vi "Updater.vi"(8 "Error In":errorcluster, 10 "This VI":refnum<vi>, 11 "Silent Error":bool) -> (0 "Error Out":errorcluster, 1 "Full command":string, 2 "File Version Info":string)   [LabVIEW 2016]
panel:
  out "standard output":string
  out "standard error":string
  out "return code":i32
  out "Application:Kind":T1(ring)
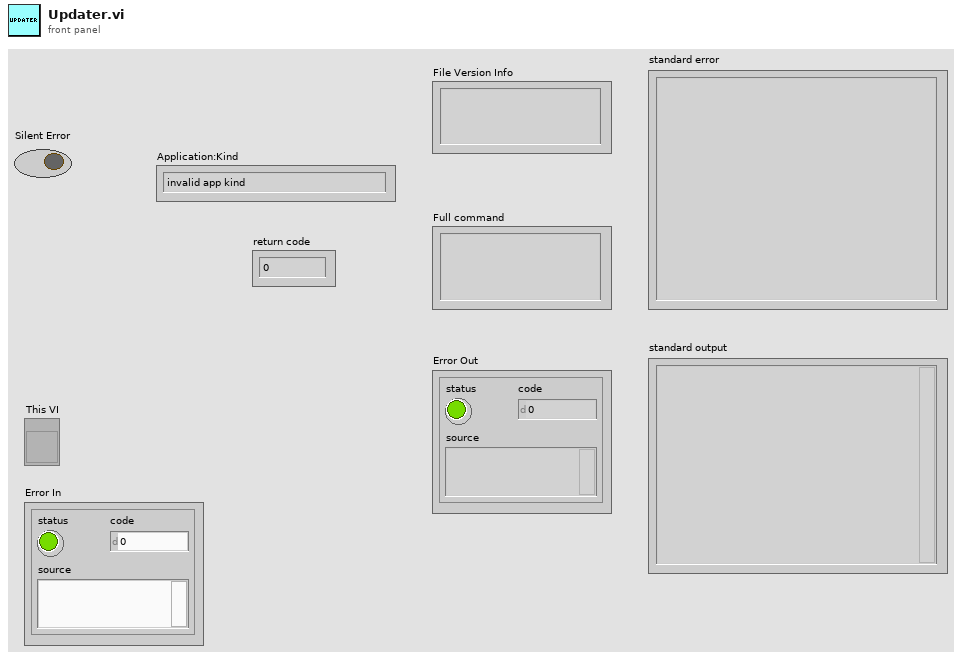
[diagram p1: front panel]
types:
  T1 = enum32{"invalid app kind", "Development System", "Run Time System", "Student Edition", "Embedded LabVIEW", "Evaluation", "Custom"}
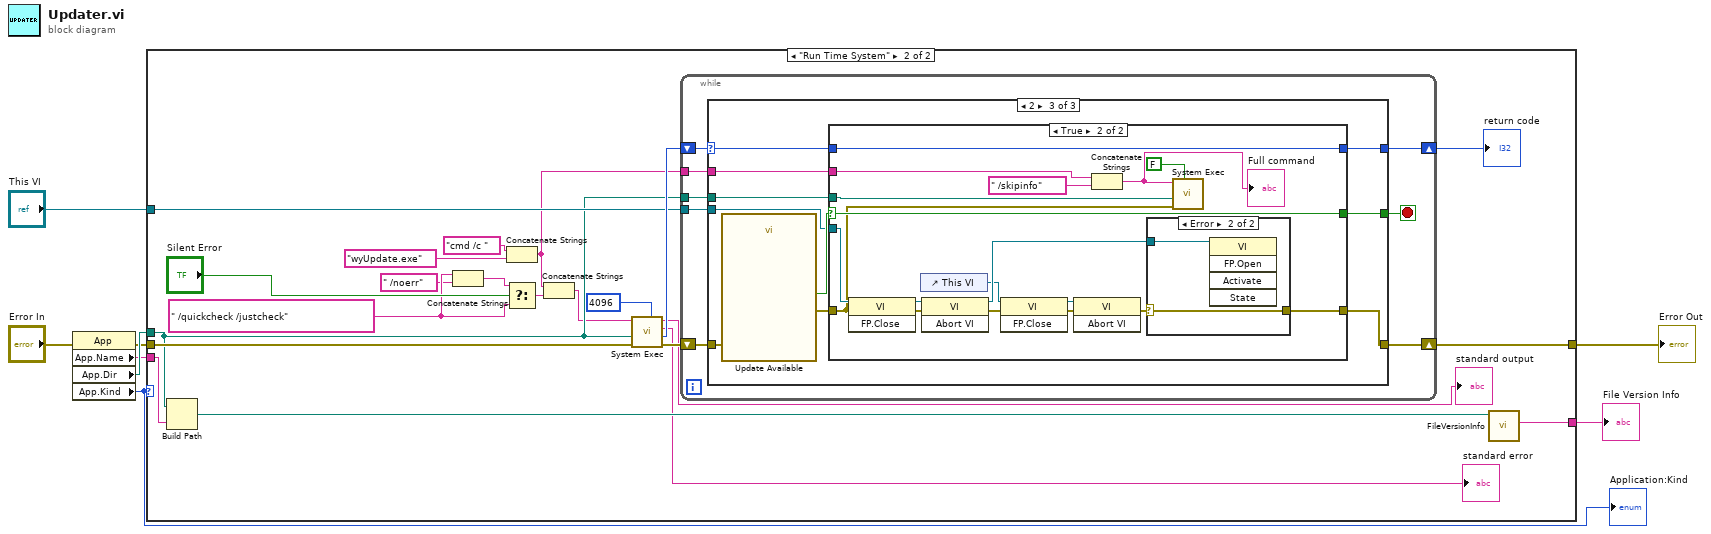
[diagram p0: block diagram]
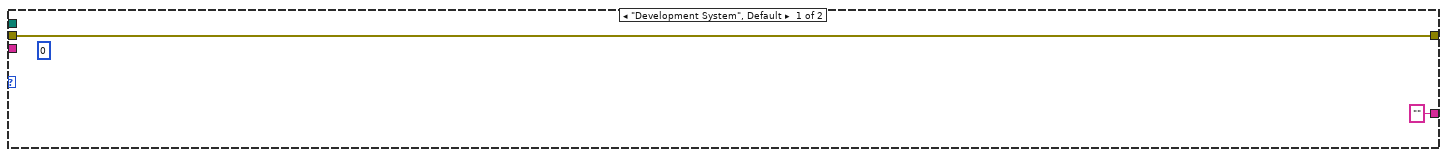
[diagram p2: hidden frame]
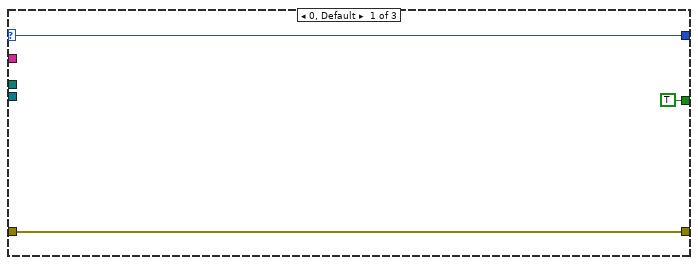
[diagram p3: hidden frame]
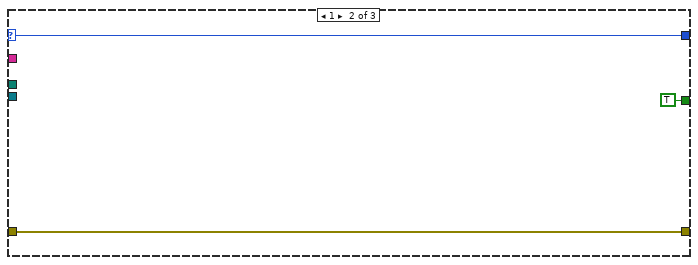
[diagram p4: hidden frame]
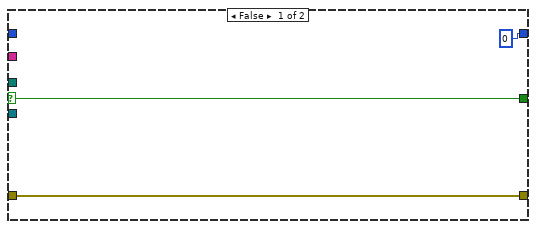
[diagram p5: hidden frame]
diagram:
  n1 = property class="App"(error in="Error In") -> (error out=w6:errorcluster, "App.Name"=w7:string, "App.Dir"=w8:path, "App.Kind"=w5:T1)  [unwired: 1 in, 1 out]
  "Application:Kind" <- w5
  n2 = case shown="\"Run Time System\"" w5 {
    tunnel: [w10 w28] -> w2
    tunnel: w6 -> [w10 w26]
    tunnel: ["" ("File Version Info") w24] -> w3
    tunnel: "This VI" -> [_ w23]
    tunnel: w7 -> [_ w22]
    tunnel: w8 -> [_ w21]
    frame "Development System", Default {
      (unwired) 0 ("return code")
    }
    frame "Run Time System" {
      w15 = " /quickcheck /justcheck" ("string")
      n3 = Build Path(base path=w21, name or relative path=w22) -> (appended path=w32:path)
      n4 = Concatenate Strings(w15, " /noerr" ("string")) -> (w16:string)
      n5 = Concatenate Strings("cmd /c " ("string"), "wyUpdate.exe" ("string")) -> (w12:string)
      n6 = Select(t=w16, s="Silent Error", f=w15) -> (s? t:f=w13:string)
      n7 = Concatenate Strings(w12, w13) -> (w11:string)
      n8 = call <vilib>:"System Exec.vi"("expected output size  (4096)"=u32 4096 ("expected output size  (4096) 2"), "error in (no error)"=w26, "working directory"=w21, "command line"=w11) -> ("error out"=w27:errorcluster, "return code"=w25:i32, "standard error"=→"standard error":string, "standard output"=→"standard output":string)  [unwired: 4 in]
      n9 = while {
        shift-right: [w36] -> w20
        shift-left: w25 -> [w40]
        tunnel: w21 -> [w38]
        tunnel: w12 -> [w37]
        shift-right: [w35] -> w28
        shift-left: w27 -> [w34]
        tunnel: w23 -> [w33]
        stop <- w39 stop-if-true
        n10 = case shown="2" w40 {
          selector: w40 -> [w42 w45 w56]
          tunnel: [TRUE TRUE w52] -> w39
          tunnel: w38 -> [_ _ w55]
          tunnel: w37 -> [_ _ w54]
          tunnel: [w42 w45 w51] -> w36
          tunnel: [w41 w44 w50] -> w35
          tunnel: w34 -> [w41 w44 w49]
          tunnel: w33 -> [_ _ w47]
          frame 0, Default {
          }
          frame 1 {
          }
          frame 2 {
            n11 = call "Update Available"("error in (no error)"=w49) -> ("OK"=w53:bool, "error out"=w48:errorcluster)  [unwired: 17 in]
            n12 = case shown="True" w53 {
              selector: w53 -> [w59 w77]
              tunnel: [w59 w77] -> w52
              tunnel: w56 -> [_ w76]
              tunnel: [0 ("return code") w76] -> w51
              tunnel: w54 -> [_ w75]
              tunnel: w48 -> [w57 w61]
              tunnel: [w57 w67] -> w50
              tunnel: w55 -> [_ w70]
              tunnel: w47 -> [_ w69]
              frame False {
              }
              frame True {
                n13 = invoke class="VI" method="FP.Close"(reference=w69, error in=w61) -> (reference out=w68:refnum<vi>, error out=w71:errorcluster)  [unwired: 1 in, 1 out]
                n14 = control-ref of="This VI"() -> (w65:refnum<vi>)
                n15 = invoke class="VI" method="Abort VI"(reference=w68, error in=w71) -> (reference out=w66:refnum<vi>, error out=w63:errorcluster)  [unwired: 1 in, 1 out]
                n16 = invoke class="VI" method="FP.Close"(reference=w65, error in=w63) -> (reference out=w64:refnum<vi>, error out=w62:errorcluster)  [unwired: 1 in, 1 out]
                n17 = invoke class="VI" method="Abort VI"(reference=w64, error in=w62) -> (error out=w60:errorcluster)  [unwired: 1 in, 2 out]
                n18 = Concatenate Strings(w75, " /skipinfo" ("string")) -> (w74:string)
                "Full command" <- w74
                n19 = case shown="Error" w60 {
                  selector: w60 -> [w78 w80]
                  tunnel: [w78 w80] -> w67
                  tunnel: w66 -> [_ w79]
                  frame No Error {
                  }
                  frame Error {
                    n20 = invoke class="VI" method="FP.Open"(reference=w79) -> ()  [unwired: 4 in, 5 out]
                  }
                }
                n21 = call <vilib>:"System Exec.vi"("wait until completion? (T)"=FALSE, "error in (no error)"=w61, "working directory"=w70, "command line"=w74) -> ()  [unwired: 4 in, 4 out]
              }
            }
          }
        }
      }
      "return code" <- w20
      n22 = call <vilib>:"FileVersionInfo.vi"("Application Path in"=w32) -> ("File Version Info"=w24:string)  [unwired: 7 in, 3 out]
    }
  }
  "File Version Info" <- w3
  "Error Out" <- w2
